vi "Run Calculator Client.vi"() -> ()   [LabVIEW 2025, in "calculator_client.lvlib"]
uses:
  calculator_client.lvlib
  RPC Messages/calculator_AddRequest.ctl
panel:
  out "error out":errorcluster
  in  "number2":dbl
  in  "number1":dbl
  out "result":dbl
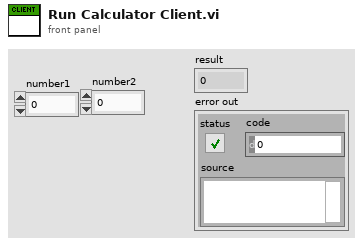
[diagram p1: front panel]
types:
  T1 = typedef "calculator_client.lvlib/calculator_AddRequest.ctl" = cluster{"number1":dbl, "number2":dbl}
  T2 = typedef "grpc-lvsupport-release.lvlib/grpcId.ctl" = u64
  T3 = typedef "calculator_client.lvlib/calculator_AddResponse.ctl" = cluster{"result":dbl}
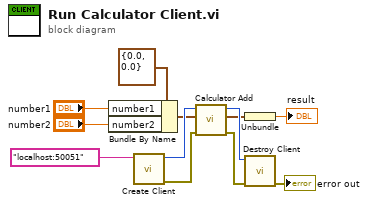
[diagram p0: block diagram]
diagram:
  n1 = Bundle By Name(cluster=T1 {"number1"=0.0, "number2"=0.0} ("Request Data"), "number1"="number1", "number2"="number2") -> (w6:T1)
  n2 = call "Create Client.vi"("address"="localhost:50051") -> ("error out"=w11:errorcluster, "gRPC ID Out"=w12:T2)  [unwired: 9 in]
  n3 = call "Calculator Add.vi"("error in"=w11, "Request Data"=w6, "gRPC ID"=w12) -> ("error out"=w9:errorcluster, "Response Data"=w5:T3, "gRPC ID out"=w10:T2)  [unwired: 6 in]
  n4 = Unbundle(w5) -> ("result"=→"result":dbl)
  n5 = call "Destroy Client.vi"("error in"=w9, "gRPC ID"=w10) -> ("error out"=→"error out":errorcluster)  [unwired: 9 in]
